vi "Inbit.vi"(0 "Strings in":string[](array[string])=["C:\\CuspControl\\GPIB and Network\\Cusp\\Inbit.txt"], 1 "Dubs in":dbl[](array[numeric])=[0.0]) -> ()   [LabVIEW 2018]
panel:
  in  "subvi":bool=TRUE
  in  "Inbit number":dbl
  in  "Inbit file":path=path "C:/CuspControl/GPIB and Network/Cusp/Inbit.txt"
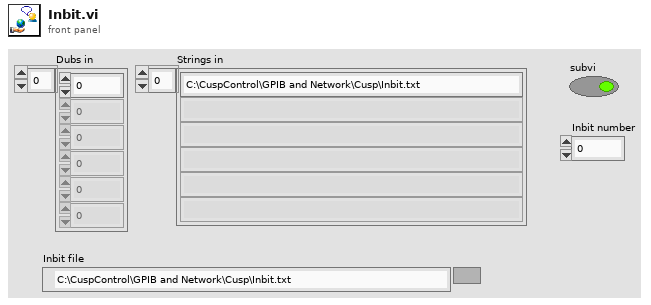
[diagram p1: front panel]
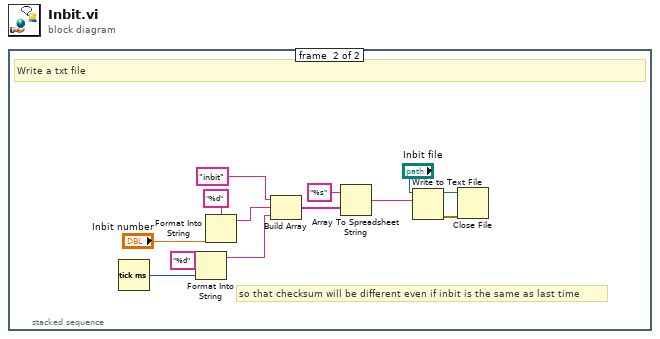
[diagram p0: block diagram]
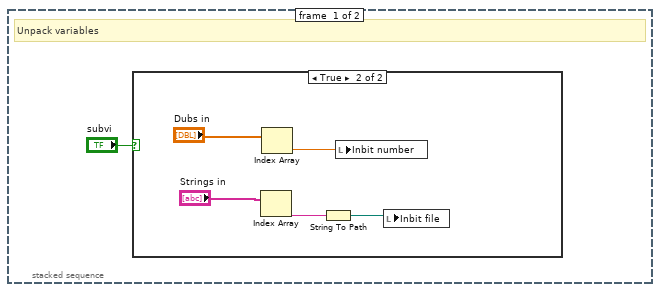
[diagram p2: hidden frame]
diagram:
  n1 = stacked-sequence {
    frame #0 {
      # "Unpack variables"
      n2 = case shown="True" "subvi" {
        frame False {
        }
        frame True {
          n3 = Index Array(array="Strings in") -> (element=w3:string)  [unwired: 1 in]
          n4 = Index Array(array="Dubs in") -> (element=w4:dbl)  [unwired: 1 in]
          n5 = String To Path(string=w3) -> (path=w2:path)
          n6 = local write "Inbit number"(w4) -> ()
          n7 = local write "Inbit file"(w2) -> ()
        }
      }
    }
    frame #1 {
      # "so that checksum will be different even if inbit is the same as last time"
      # "Write a txt file"
      n8 = Tick Count (ms)() -> (millisecond timer value=w8:u32)
      n9 = Format Into String(format string="%d", w8) -> (resulting string=w7:string)  [unwired: 2 in, 1 out]
      n10 = Format Into String(format string="%d", "Inbit number") -> (resulting string=w11:string)  [unwired: 2 in, 1 out]
      n11 = Build Array("inbit" ("format string"), w11, w7) -> (w10:string[])
      n12 = Array To Spreadsheet String(array=w10, 3:"%s" ("format string")) -> (spreadsheet string=w14:string)  [unwired: 1 in]
      n13 = Write to Text File(file (use dialog)="Inbit file", text=w14) -> (refnum out=w15:refnum<file>, error out=w16:errorcluster)  [unwired: 2 in, 1 out]
      n14 = Close File(refnum=w15, error in=w16) -> ()  [unwired: 2 out]
    }
  }
